vi "CreatePublicEvents.vi"(8 "error in (no error)":errorcluster, 11 "LockinDAQ":refnum<class "Lockin.DAQ.lvclass">=refnum) -> (0 "error out":errorcluster, 3 "LockinDAQ out":refnum<class "Lockin.DAQ.lvclass">)   [LabVIEW 2016, in "Lockin.DAQ.lvclass"]
doc: "---------------------------------------------------------------\nJKI State Machine Objects™\nhttp://jki.net/state-machine-objects/\nCopyright (C) 2005-2015, JKI <info@jki.net>\nALL RIGHTS RESERVEDJKI State Machine Objects (SMO) 1.0.0.4\nJKI - JKI\nCopyright (c) 2015, JKI"
uses:
  Lockin.DAQ.lvclass
  Typedefs/PublicEvents--Lockin.DAQ.getAO.ctl
  Typedefs/PublicEvents--Lockin.DAQ.getAI.ctl
  Typedefs/PublicEvents--Lockin.DAQ.getREF.ctl
  Typedefs/PublicEvents--Lockin.DAQ.getResults.ctl
  Typedefs/Results--Cluster.ctl
  Typedefs/PublicEvents--Lockin.DAQ.getCalibration.ctl
  Typedefs/Cal Info - Cluster.ctl
  Typedefs/PublicEvents--Lockin.DAQ.getAOChannels.ctl
  Typedefs/AO-cluster.ctl
  Typedefs/Function-enum.ctl
  Typedefs/PublicEvents--Lockin.DAQ.getREFChannels.ctl
  Typedefs/REF-cluster.ctl
  Typedefs/PublicEvents--Lockin.DAQ.getDAQState.ctl
  Typedefs/State-enum.ctl
  Typedefs/PublicEvents--Lockin.DAQ.getSweepResults.ctl
  Typedefs/SweepResults--Cluster.ctl
  Typedefs/PublicEvents--Lockin.DAQ.getSweepWaveforms.ctl
  Typedefs/PublicEvents--Lockin.DAQ.getDAQconfig.ctl
  Typedefs/New Channel Cluster.ctl
  Typedefs/446xAI-enum.ctl
  Typedefs/AI.coupling-enum.ctl
  Typedefs/446xAO-enum.ctl
  Lockin.DAQ.lvclass/Lockin.DAQ.ctl
  <vilib>/JKI/JKI SMO/SMO/SMO.lvclass
panel:
  # "For instructions on how to use the JKI State Machine Objects, examples and video tutorials, visit:\nhttp://jki.net/state-machine-objects/\n\nJKI State Machine Objects™\nhttp://jki.net/state-machine-objects/\nCopyright (C) 2005-2015, JKI <info@jki.net>\nALL RIGHTS RESERVED"
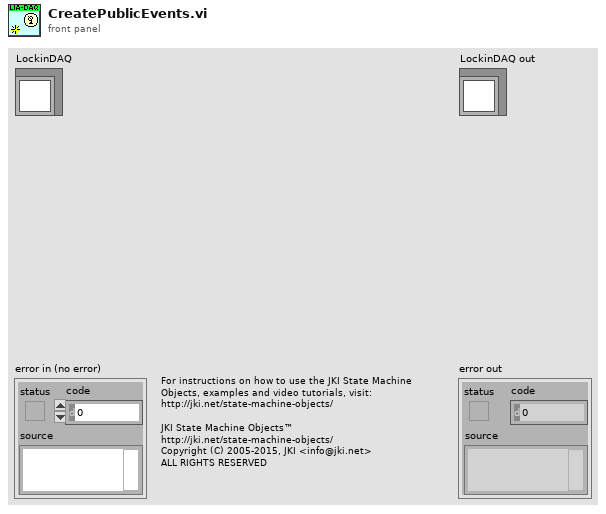
[diagram p1: front panel]
types:
  T1 = typedef "Lockin.DAQ.lvclass/PublicEvents--Lockin.DAQ.getDAQconfig.ctl" = T2[]
  T2 = typedef "Lockin.DAQ.lvclass/New Channel Cluster.ctl" = cluster{"Device":string, "AI.Ch":string, "AI.Range":T3, "AI.Coupling":T4, "AO.Ch":string, "AO.Range":T5, "LIA.Ch":string}
  T3 = typedef "Lockin.DAQ.lvclass/446xAI-enum.ctl" = enum16{"±0.316 V", "±1.00 V", "±3.16 V", "±10.0 V", "±31.6 V", "±42.4 V"}
  T4 = typedef "Lockin.DAQ.lvclass/AI.coupling-enum.ctl" = u16
  T5 = typedef "Lockin.DAQ.lvclass/446xAO-enum.ctl" = enum16{"±0.1 V", "±1.0 V", "±10.0 V"}
  T6 = typedef "Lockin.DAQ.lvclass/PublicEvents--Lockin.DAQ.getSweepWaveforms.ctl" = cluster{"Sweep_AO":waveform(dbl)[], "Sweep_AI":waveform(dbl)[]}
  T7 = typedef "Lockin.DAQ.lvclass/PublicEvents--Lockin.DAQ.getSweepResults.ctl" = cluster{"getSweepResults":T8}
  T8 = typedef "Lockin.DAQ.lvclass/SweepResults--Cluster.ctl" = cluster{"Time Stamp":timestamp, "X Results":cluster{"parameter":dbl[], "x":dbl[]}[], "Y Results":cluster{"parameter":dbl[], "y":dbl[]}[]}
  T9 = typedef "Lockin.DAQ.lvclass/PublicEvents--Lockin.DAQ.getDAQState.ctl" = cluster{"state":T10}
  T10 = typedef "Lockin.DAQ.lvclass/State-enum.ctl" = enum16{"idle", "created", "started", "stopped", "sweeping"}
  T11 = typedef "Lockin.DAQ.lvclass/PublicEvents--Lockin.DAQ.getREFChannels.ctl" = cluster{"Channels: REF":T12}
  T12 = typedef "Lockin.DAQ.lvclass/REF-cluster.ctl" = cluster{"Ch":i32[], " f (Hz)":dbl[], "Phase (°)":dbl[], "TC (s)":dbl[], "order":i32[]}
  T13 = typedef "Lockin.DAQ.lvclass/PublicEvents--Lockin.DAQ.getAOChannels.ctl" = cluster{"Channels: AO":T14}
  T14 = typedef "Lockin.DAQ.lvclass/AO-cluster.ctl" = cluster{"Ch":i32[], "Amp (V)":dbl[], "DC (V)":dbl[], "f (Hz)":dbl[], "Phase (°)":dbl[], "Function":T15[], "Sweep?":bool[]}
  T15 = typedef "Lockin.DAQ.lvclass/Function-enum.ctl" = enum16{"Sine", "Triangle", "Square", "Sawtooth"}
  T16 = typedef "Lockin.DAQ.lvclass/PublicEvents--Lockin.DAQ.getCalibration.ctl" = T17[]
  T17 = typedef "Lockin.DAQ.lvclass/Cal Info - Cluster.ctl" = cluster{"Active Device":string, "SelfCal.LastDate/Time":dbl, "SelfCal.LastTemp":dbl, "DevTemp":dbl, "calibration due?":bool}
  T18 = typedef "Lockin.DAQ.lvclass/PublicEvents--Lockin.DAQ.getResults.ctl" = cluster{"Results":T19}
  T19 = typedef "Lockin.DAQ.lvclass/Results--Cluster.ctl" = cluster{"Time Stamp":timestamp, "Results":dbl[][]}
  T20 = typedef "Lockin.DAQ.lvclass/PublicEvents--Lockin.DAQ.getREF.ctl" = waveform(dbl)[]
  T21 = typedef "Lockin.DAQ.lvclass/PublicEvents--Lockin.DAQ.getAI.ctl" = waveform(dbl)[]
  T22 = typedef "Lockin.DAQ.lvclass/PublicEvents--Lockin.DAQ.getAO.ctl" = waveform(dbl)[]
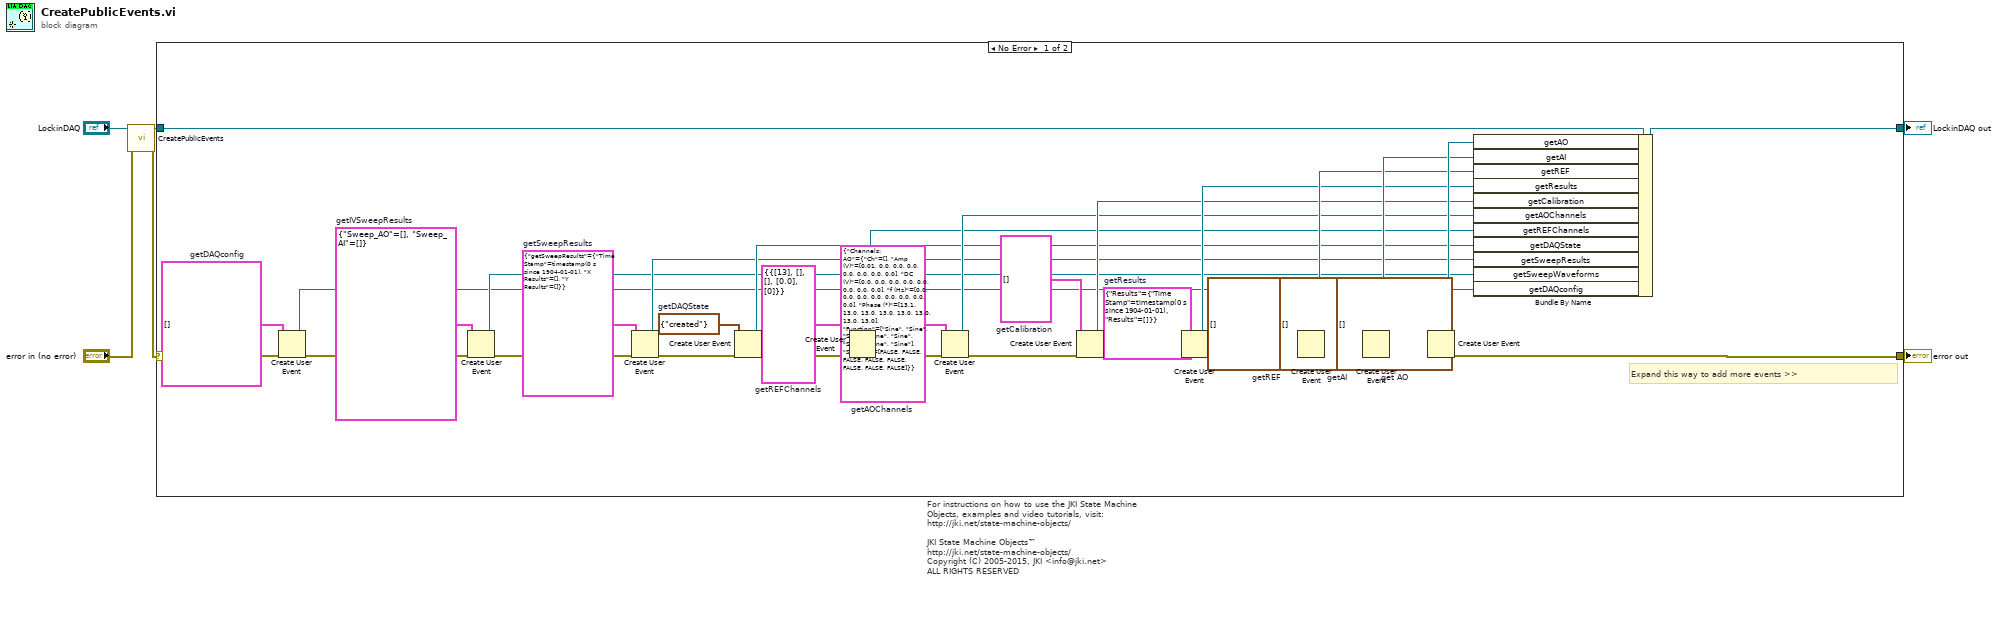
[diagram p0: block diagram]
diagram:
  # "For instructions on how to use the JKI State Machine Objects, examples and video tutorials, visit:\nhttp://jki.net/state-machine-objects/\n\nJKI State Machine Objects™\nhttp://jki.net/state-machine-objects/\nCopyright (C) 2005-2015, JKI <info@jki.net>\nALL RIGHTS RESERVED"
  n1 = call-parent "CreatePublicEvents.vi"("error in (no error)"="error in (no error)", "SMO"="LockinDAQ") -> ("error out"=w1:errorcluster, "SMO out"=w3:refnum<class "Lockin.DAQ.lvclass">)  [unwired: 8 in]
  n2 = case shown="No Error" w1 {
    selector: w1 -> [w41 w44]
    tunnel: [w39 w44] -> w5
    tunnel: [w40 w43] -> w6
    tunnel: w3 -> [w42 w43]
    frame No Error {
      w8 = T1 []  # getDAQconfig
      w11 = T6 {"Sweep_AO"=[], "Sweep_AI"=[]}  # getIVSweepResults
      w14 = T7 {"getSweepResults"={"Time Stamp"=timestamp(0 s since 1904-01-01), "X Results"=[], "Y Results"=[]}}  # getSweepResults
      w17 = T9 {"state"=enum."created"}  # getDAQState
      w20 = T11 {"Channels: REF"={"Ch"=[13], " f (Hz)"=[], "Phase (°)"=[], "TC (s)"=[0.0], "order"=[0]}}  # getREFChannels
      w23 = T13 {"Channels: AO"={"Ch"=[], "Amp (V)"=[0.01, 0.0, 0.0, 0.0, 0.0, 0.0, 0.0, 0.0], "DC (V)"=[0.0, 0.0, 0.0, 0.0, 0.0, 0.0, 0.0, 0.0], "f (Hz)"=[0.0, 0.0, 0.0, 0.0, 0.0, 0.0, 0.0, 0.0], "Phase (°)"=[13.1, 13.0, 13.0, 13.0, 13.0, 13.0, 13.0, 13.0], "Function"=[enum."Sine", enum."Sine", enum."Sine", enum."Sine", enum."Sine", enum."Sine", enum."Sine", enum."Sine"], "Sweep?"=[FALSE, FALSE, FALSE, FALSE, FALSE, FALSE, FALSE, FALSE]}}  # getAOChannels
      w26 = T16 []  # getCalibration
      w29 = T18 {"Results"={"Time Stamp"=timestamp(0 s since 1904-01-01), "Results"=[]}}  # getResults
      w32 = T20 []  # getREF
      w35 = T21 []  # getAI
      w38 = T22 []  # get AO
      # "Expand this way to add more events >>"
      n3 = Create User Event(user event datatype=w8, error in=w41) -> (user event=w7:refnum<user-event>, error out=w9:errorcluster)
      n4 = Create User Event(user event datatype=w11, error in=w9) -> (user event=w10:refnum<user-event>, error out=w12:errorcluster)
      n5 = Create User Event(user event datatype=w14, error in=w12) -> (user event=w13:refnum<user-event>, error out=w15:errorcluster)
      n6 = Create User Event(user event datatype=w17, error in=w15) -> (user event=w16:refnum<user-event>, error out=w18:errorcluster)
      n7 = Create User Event(user event datatype=w20, error in=w18) -> (user event=w19:refnum<user-event>, error out=w21:errorcluster)
      n8 = Create User Event(user event datatype=w23, error in=w21) -> (user event=w22:refnum<user-event>, error out=w24:errorcluster)
      n9 = Create User Event(user event datatype=w26, error in=w24) -> (user event=w25:refnum<user-event>, error out=w27:errorcluster)
      n10 = Create User Event(user event datatype=w29, error in=w27) -> (user event=w28:refnum<user-event>, error out=w30:errorcluster)
      n11 = Create User Event(user event datatype=w32, error in=w30) -> (user event=w31:refnum<user-event>, error out=w33:errorcluster)
      n12 = Create User Event(user event datatype=w35, error in=w33) -> (user event=w34:refnum<user-event>, error out=w36:errorcluster)
      n13 = Create User Event(user event datatype=w38, error in=w36) -> (user event=w37:refnum<user-event>, error out=w39:errorcluster)
      n14 = Bundle By Name(cluster=w42, "getAO"=w37, "getAI"=w34, "getREF"=w31, "getResults"=w28, "getCalibration"=w25, "getAOChannels"=w22, "getREFChannels"=w19, "getDAQState"=w16, "getSweepResults"=w13, "getSweepWaveforms"=w10, "getDAQconfig"=w7) -> (w40:refnum<class "Lockin.DAQ.lvclass">)
    }
    frame Error {
    }
  }
  "error out" <- w5
  "LockinDAQ out" <- w6
